vi "Create Registered Channel Types.vi"(8 "error in":errorcluster, 11 "Channel Definition in":T1 {"Custom Config Data" format="%x"}) -> (0 "error out":errorcluster, 1 "Not Registered":bool, 2 "Channel out":refnum<class "CIFChannels.lvclass">, 3 "Channel Definition out":T1 {"Custom Config Data" format="%x"})   [LabVIEW 2021, in "ChannelRegistrar.lvlib"]
uses:
  ChannelRegistrar.lvlib
  typedef/Channel Definition.ctl
  <vilib>/CIF Foundation/CIF Channels Core/CIFChannels/Typedef/Direction.ctl
  typedef/Registered Channel Types.ctl
  <vilib>/CIF Foundation/CIF Channels Core/CIFChannels/CIFChannels.lvclass
  <vilib>/CIF Foundation/CIF Channels Core/CIF_NIChn/Double/CIF_NIChn_Double.lvclass
  C:/Program Files/National Instruments/LabVIEW 2021/vi.lib/CIF Foundation/CIF Channels Core/CIFChannels/CIFChannels.lvclass
  <vilib>/CIF Foundation/CIF Channels Core/CIF_NIChn/U64/CIF_NIChn_U64.lvclass
  <vilib>/CIF Foundation/CIF Channels Core/CIF_NIChn/I64/CIF_NIChn_I64.lvclass
  <vilib>/CIF Foundation/CIF Channels Core/CIF_NIChn/FIFO_RAW/CIF_NIChn_Raw.lvclass
  <vilib>/CIF Foundation/CIF Channels Core/CIF_NIChn/FIFO_CAN/CIF_NIChn_CAN.lvclass
  <vilib>/CIF Foundation/CIF Channels Core/CIF_NIChn/FIFO_L2Enet/CIF_NIChn_L2Enet.lvclass
  <vilib>/CIF Foundation/CIF Channels Core/CIF_NIChn/FIFO_DAQ/CIF_NIChn_DAQ.lvclass
  C:/Program Files/National Instruments/LabVIEW 2021/vi.lib/CIF Foundation/CIF Channels Core/CIF_NIChn/FIFO_U8_Multi/CIF_Fifo_U8_Multi.lvclass
  C:/Program Files/National Instruments/LabVIEW 2021/vi.lib/CIF Foundation/CIF Channels Core/CIF_NIChn/FIFO_U8/CIF_NIChn_Fifo_U8.lvclass
  C:/Program Files/National Instruments/LabVIEW 2021/vi.lib/CIF Foundation/CIF Channels Core/CIF_NIChn/NIChn/CIF_NIChn.lvclass
  C:/Program Files/National Instruments/LabVIEW 2021/vi.lib/CIF Foundation/CIF Channels Core/CIF_NIChn/FIFO_CAN/CIF_NIChn_CAN.lvclass
  C:/Program Files/National Instruments/LabVIEW 2021/vi.lib/CIF Foundation/CIF Channels Core/CIF_NIChn/FIFO_L2Enet/CIF_NIChn_L2Enet.lvclass
  C:/Program Files/National Instruments/LabVIEW 2021/vi.lib/CIF Foundation/CIF Channels Core/CIF_NIChn/FIFO_DAQ/DAQ Base/CIF_NIChn_DAQ_Base.lvclass
  C:/Program Files/National Instruments/LabVIEW 2021/vi.lib/CIF Foundation/CIF Channels Core/CIF_NIChn/FIFO_DAQ/CIF_NIChn_DAQ.lvclass
  <vilib>/CIF Foundation/CIF Channels Core/CIPC_Channels/Double/CIF_CIPC_Chn_Double.lvclass
  <vilib>/CIF Foundation/CIF Channels Core/CIPC_Channels/U64/CIF_CIPC_Chn_U64.lvclass
  <vilib>/CIF Foundation/CIF Channels Core/CIPC_Channels/I64/CIF_CIPC_Chn_I64.lvclass
  C:/Program Files/National Instruments/LabVIEW 2021/vi.lib/CIF Foundation/CIF Channels Core/CIPC_Channels/CIF_CIPC_Chan/CIF_CIPC_Chn.lvclass
  C:/Program Files/National Instruments/LabVIEW 2021/vi.lib/CIF Foundation/CIF Channels Core/CIPC_Channels/Double/CIF_CIPC_Chn_Double.lvclass
  C:/Program Files/National Instruments/LabVIEW 2021/vi.lib/CIF Foundation/CIF Channels Core/CIPC_Channels/I64/CIF_CIPC_Chn_I64.lvclass
  C:/Program Files/National Instruments/LabVIEW 2021/vi.lib/CIF Foundation/CIF Channels Core/CIPC_Channels/U64/CIF_CIPC_Chn_U64.lvclass
  C:/Program Files/National Instruments/LabVIEW 2021/vi.lib/CIF Foundation/CIF Channels Core/CIF_NIChn/Double/CIF_NIChn_Double.lvclass
  C:/Program Files/National Instruments/LabVIEW 2021/vi.lib/CIF Foundation/CIF Channels Core/CIF_NIChn/U64/CIF_NIChn_U64.lvclass
  C:/Program Files/National Instruments/LabVIEW 2021/vi.lib/CIF Foundation/CIF Channels Core/CIF_NIChn/I64/CIF_NIChn_I64.lvclass
  C:/Program Files/National Instruments/LabVIEW 2021/vi.lib/CIF Foundation/CIF Channels Core/CIF_NIChn/FIFO_RAW/CIF_NIChn_Raw.lvclass
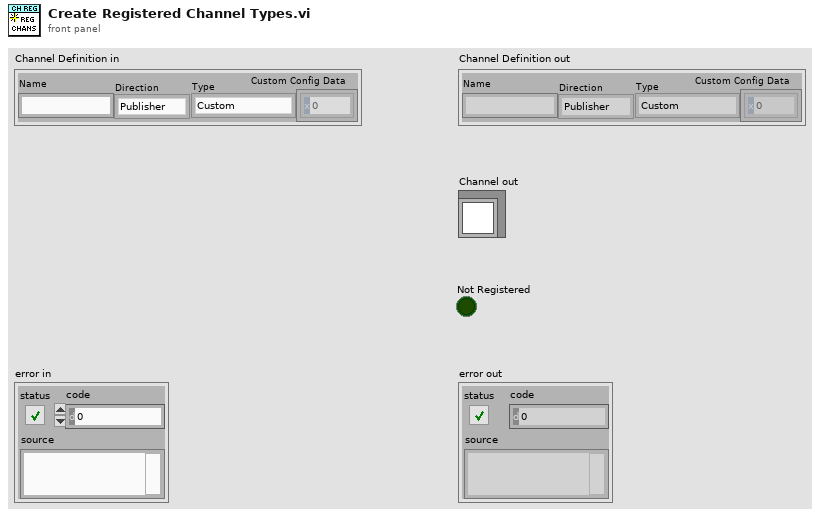
[diagram p1: front panel]
types:
  T1 = typedef "ChannelRegistrar.lvlib/Channel Definition.ctl" = cluster{"Name":string, "Direction":T2, "Type":T3, "Custom Config Data":u8[]}
  T2 = typedef "CIFChannels.lvclass/Direction.ctl" = enum16{"Publisher", "Subscriber"}
  T3 = typedef "ChannelRegistrar.lvlib/Registered Channel Types.ctl" = enum16{"Custom", "CIF_CIPC_Double", "CIF_CIPC_I64", "CIF_CIPC_U64", "CIF_NIChn_Double", "CIF_NIChn_I64", "CIF_NIChn_U64", "CIF_NIChn_Raw", "CIF_NIChn_CAN", "CIF_NIChn_L2Enet", "CIF_NIChn_DAQ"}
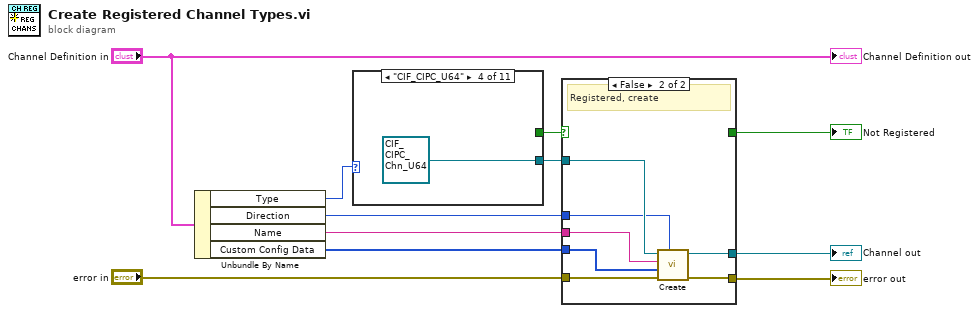
[diagram p0: block diagram]
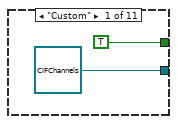
[diagram p2: hidden frame]
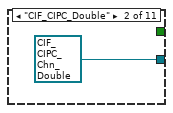
[diagram p3: hidden frame]
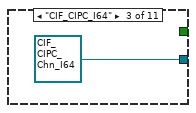
[diagram p4: hidden frame]
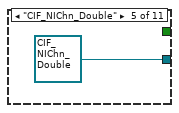
[diagram p5: hidden frame]
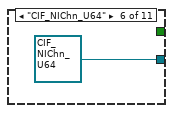
[diagram p6: hidden frame]
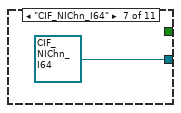
[diagram p7: hidden frame]
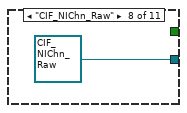
[diagram p8: hidden frame]
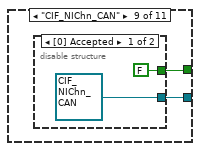
[diagram p9: hidden frame]
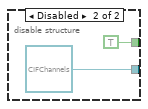
[diagram p10: hidden frame]
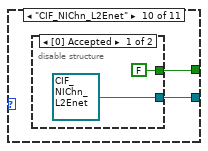
[diagram p11: hidden frame]
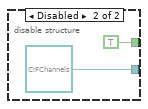
[diagram p12: hidden frame]
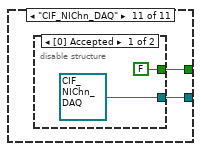
[diagram p13: hidden frame]
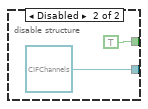
[diagram p14: hidden frame]
diagram:
  n1 = Unbundle By Name("Channel Definition in") -> ("Type"=w1:T3, "Direction"=w11:T2, "Name"=w10:string, "Custom Config Data"=w9:u8[])
  n2 = case shown="\"CIF_CIPC_U64\"" w1 {
    tunnel: [TRUE _ _ _ _ _ _ _ w21 w27 w33] -> w4
    tunnel: [refnum<class "CIFChannels.lvclass"> refnum ("Channel out 2") refnum<class "CIF_CIPC_Chn_Double.lvclass"> refnum ("CIF_CIPC_Chn_Double.lvclass") refnum<class "CIF_CIPC_Chn_I64.lvclass"> refnum ("CIF_CIPC_Chn_I64.lvclass") refnum<class "CIF_CIPC_Chn_U64.lvclass"> refnum ("CIF_CIPC_Chn_U64.lvclass") refnum<class "CIF_NIChn_Double.lvclass"> refnum ("CIFTagDouble.lvclass") refnum<class "CIF_NIChn_U64.lvclass"> refnum ("CIFTagU64.lvclass") refnum<class "CIF_NIChn_I64.lvclass"> refnum ("CIFTagI64.lvclass") refnum<class "CIF_NIChn_Raw.lvclass"> refnum ("CIF_Fifo_Raw_Multi in") w22 w28 w34] -> w3
    frame "Custom" {
    }
    frame "CIF_CIPC_Double" {
    }
    frame "CIF_CIPC_I64" {
    }
    frame "CIF_CIPC_U64" {
    }
    frame "CIF_NIChn_Double" {
    }
    frame "CIF_NIChn_U64" {
    }
    frame "CIF_NIChn_I64" {
    }
    frame "CIF_NIChn_Raw" {
    }
    frame "CIF_NIChn_CAN" {
      n3 = disable-structure shown="[0] Accepted" {
        disable-tunnel: [refnum<class "CIF_NIChn_CAN.lvclass"> refnum ("CIF_NIChn_CAN.lvclass") refnum<class "CIFChannels.lvclass"> refnum ("Channel out 2")] -> w22
        disable-tunnel: [FALSE TRUE] -> w21
        frame Enabled {
        }
        frame Disabled {
        }
      }
    }
    frame "CIF_NIChn_L2Enet" {
      n4 = disable-structure shown="[0] Accepted" {
        disable-tunnel: [refnum<class "CIF_NIChn_L2Enet.lvclass"> refnum ("CIF_NIChn_L2Enet.lvclass") refnum<class "CIFChannels.lvclass"> refnum ("Channel out 2")] -> w28
        disable-tunnel: [FALSE TRUE] -> w27
        frame Enabled {
        }
        frame Disabled {
        }
      }
    }
    frame "CIF_NIChn_DAQ" {
      n5 = disable-structure shown="[0] Accepted" {
        disable-tunnel: [refnum<class "CIF_NIChn_DAQ.lvclass"> refnum ("CIF_NIChn_DAQ.lvclass") refnum<class "CIFChannels.lvclass"> refnum ("Channel out 2")] -> w34
        disable-tunnel: [FALSE TRUE] -> w33
        frame Enabled {
        }
        frame Disabled {
        }
      }
    }
  }
  n6 = case shown="False" w4 {
    selector: w4 -> [w39 _]
    tunnel: w11 -> [_ w44]
    tunnel: w10 -> [_ w43]
    tunnel: w9 -> [_ w42]
    tunnel: "error in" -> [w40 w46]
    tunnel: [w40 w45] -> w7
    tunnel: [_ w41] -> w2
    tunnel: [w39 _] -> w5
    tunnel: w3 -> [_ w47]
    frame True {
      # "Not registered"
    }
    frame False {
      # "Registered, create"
      n7 = call-dynamic "Create.vi"("Direction"=w44, "error in (no error)"=w46, "Custom Config Data"=w42, "Name"=w43, "CIFChannels in"=w47) -> ("error out"=w45:errorcluster, "CIFChannels out"=w41:refnum<class "CIFChannels.lvclass">)  [unwired: 5 in]
    }
  }
  "error out" <- w7
  "Channel out" <- w2
  "Not Registered" <- w5
  "Channel Definition out" <- "Channel Definition in"
